vi "water indicate.vi"() -> ()   [LabVIEW 2020]
panel:
  in  "stop":bool
  out "Boolean 2":bool
  out "Boolean":bool
  out "Tank":dbl(slide) scale=0.0..10.0
  in  "Numeric":dbl
  # "WATER LEVEL  INDICATOR"
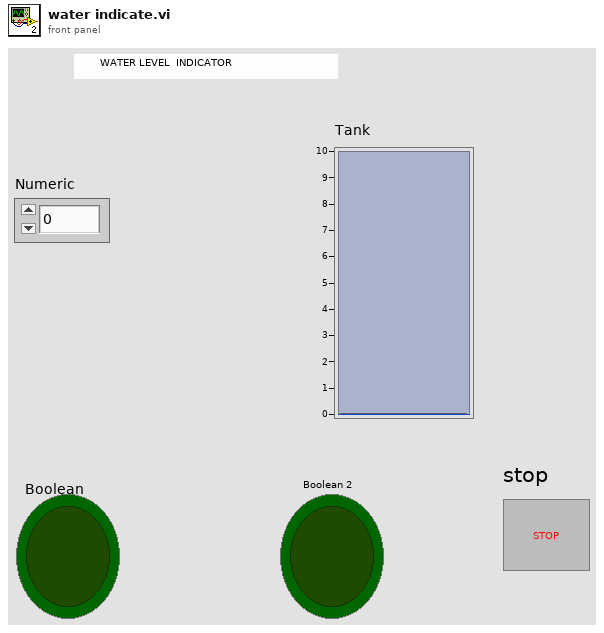
[diagram p1: front panel]
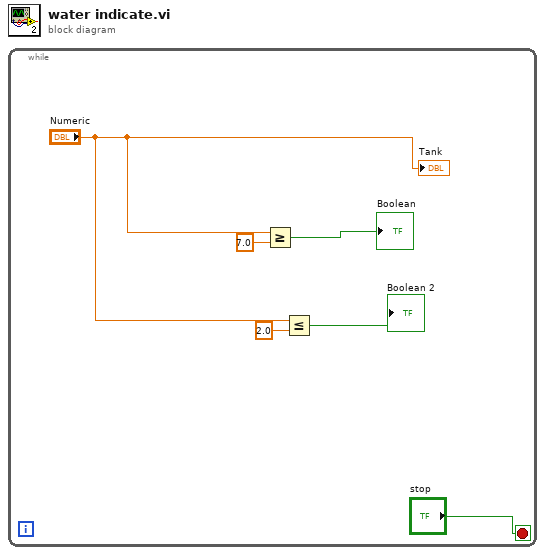
[diagram p0: block diagram]
diagram:
  n1 = while {
    stop <- "stop" stop-if-true
    n2 = Greater Or Equal?(x="Numeric", y=7.0) -> (x >= y?=→"Boolean":bool)
    n3 = Less Or Equal?(x="Numeric", y=2.0) -> (x <= y?=→"Boolean 2":bool)
    "Tank" <- "Numeric"
  }
